vi "Begin.vi"(8 "error in":errorcluster) -> (0 "error out":errorcluster)   [LabVIEW 2020]
doc: "Called before other user functions, this VI is expected to open initial I/O refnums, load in file data, and do all program initialization. Notice that the <B>error out</B> terminal is simply used for data flow. Wiring it to other structures or subVIs ensures that this VI runs first."
uses:
  <vilib>/Rock Robotics/WPI/DriverStation/WPI_DriverStationRobotMode2.ctl
  <vilib>/Rock Robotics/WPI/Joystick/WPI_JoystickDeviceEnum.ctl
  <vilib>/Rock Robotics/SystemInterfaces/i2clib/i2c_bus.ctl
  <vilib>/Rock Robotics/WPI/Solenoid/WPI_SolenoidChannel.ctl
  <vilib>/Rock Robotics/SystemInterfaces/DIO/FPGA_DIOChannel.ctl
  <vilib>/Rock Robotics/WPI/ThirdParty/Phoenix-LabVIEW/Motor Controller/Controls/CTRE_Phoenix_MotorControl_StatusFrameEnhanced.ctl
  Robot Global Data.vi
  <vilib>/Rock Robotics/Network Tables/NT Write String Array.vi
  <vilib>/Rock Robotics/WPI/Solenoid/WPI_SolenoidOpenDouble.vi
  <vilib>/Rock Robotics/WPI/Switch/WPI_SwitchOpenLimit.vi
  <vilib>/Rock Robotics/WPI/Switch/WPI_SwitchOpenCounting.vi
  <vilib>/Rock Robotics/WPI/ThirdParty/Phoenix-LabVIEW/Motor Controller/Get/CTRE_Phoenix_MotorController_GetSelectedSensorData.vi
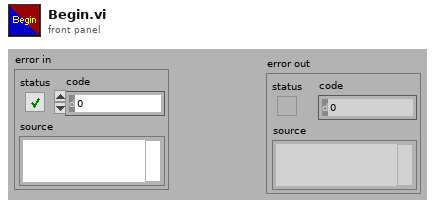
[diagram p1: front panel]
types:
  T1 = typedef "CTRE_Phoenix_MotorControl_StatusFrameEnhanced.ctl" = u16
  T2 = typedef "FPGA_DIOChannel.ctl" = enum8{"DIO 0", "DIO 1", "DIO 2", "DIO 3", "DIO 4", "DIO 5", "DIO 6", "DIO 7", "DIO 8", "DIO 9", "DIO MXP 0", "DIO MXP 1", "DIO MXP 2", "DIO MXP 3", "DIO MXP 4", "DIO MXP 5", "DIO MXP 6", "DIO MXP 7", "DIO MXP 8", "DIO MXP 9", "DIO MXP 10", "DIO MXP 11", "DIO MXP 12", "DIO MXP 13", "DIO MXP 14", "DIO MXP 15", "SPI Port CS1", "SPI Port CS2", "SPI Port CS3", "SPI Port MISO", "SPI Port MOSI", "Invalid"}
  T3 = typedef "WPI_SolenoidChannel.ctl" = enum8{"Solenoid 0", "Solenoid 1", "Solenoid 2", "Solenoid 3", "Solenoid 4", "Solenoid 5", "Solenoid 6", "Solenoid 7", "Solenoid 8", "Solenoid 9", "Solenoid 10", "Solenoid 11", "Solenoid 12", "Solenoid 13", "Solenoid 14", "Solenoid 15", "Invalid"}
  T4 = typedef "i2c_bus.ctl" = enum16{"I2C On-Board", "I2C MXP", "Invalid"}
  T5 = typedef "WPI_JoystickDeviceEnum.ctl" = enum16{"USB 0", "USB 1", "USB 2", "USB 3", "USB 4", "USB 5"}
  T6 = typedef "WPI_DriverStationRobotMode2.ctl" = enum16{"Autonomous Disabled", "Autonomous Enabled", "Teleop Disabled", "Teleop Enabled", "Disconnected", "Finish", "Test Disabled", "Test Enabled", "Emergency Stopped"}
  T7 = typedef "WPI_JoystickDevRef.ctl" = cluster{"Device":T5}
  T8 = typedef "WPI_CompressorDevRef.ctl" = cluster{"DevStatus":errorcluster, "Pneumatics Control Module":u8}
  T9 = typedef "WPI_SolenoidDevRef.ctl" = cluster{"DevStatus":errorcluster, "Pneumatics Control Module":u8, "Forward Solenoid Channel":T3, "Reverse Solenoid Channel":T3}
  T10 = typedef "WPI_SwitchDevRef.ctl" = cluster{"DevStatus":errorcluster, "DIO Channel":T2, "CntIndex":T11, "Normally Closed":bool}
  T11 = typedef "FPGA_CounterCtrSystemIndex.ctl" = enum8{"Ctr 0", "Ctr 1", "Ctr 2", "Ctr 3", "Ctr 4", "Ctr 5", "Ctr 6", "Ctr 7", "Invalid"}
  T12 = typedef "WPI_MotorControlDeviceRef.ctl" = cluster{"DeviceStatus":errorcluster, "Type":T13, "PWM":cluster{"PWM Channel":T14, "DeadBand":T15}, "CAN":cluster{"Device Number":u8, "SetOutput VI Ref":variant, "GetOutput VI Ref":variant, "Enable VI Ref":variant, "Disable VI Ref":variant, "Data":variant}, "Invert":bool, "DIO PWM":cluster{"PWM \"Enable\" Channel":T14, "DIOChannel":T2, "PWM Rate":dbl}}
  T13 = typedef "WPI_MotorControlType.ctl" = enum16{"PWM", "CAN", "DIO PWM"}
  T14 = typedef "FPGA_DIOPWMChannel.ctl" = enum8{"PWM 0", "PWM 1", "PWM 2", "PWM 3", "PWM 4", "PWM 5", "PWM 6", "PWM 7", "PWM 8", "PWM 9", "PWM MXP 0", "PWM MXP 1", "PWM MXP 2", "PWM MXP 3", "PWM MXP 4", "PWM MXP 5", "PWM MXP 6", "PWM MXP 7", "PWM MXP 8", "PWM MXP 9", "Invalid"}
  T15 = typedef "WPI_PWMDeadband.ctl" = cluster{"Name":string, "maxPositivePwm":i32, "minPositivePwm":i32, "centerPwm":i32, "maxNegativePwm":i32, "minNegativePwm":i32, "angularRange":u16}
  T16 = typedef "Color Sensor V3 DevRef.ctl" = cluster{"I2CDevRef":T17}
  T17 = typedef "WPI_I2CDevRef.ctl" = cluster{"DevStatus":errorcluster, "Device Address":u8, "Handle":i32, "I2C Bus":T4}
  T18 = typedef "CTRE_PigeonIMU_DeviceRef.ctl" = cluster{"DeviceStatus":errorcluster, "Device Number":u8, "Type":T19, "Device ID":u32, "Handle":u64, "UsageFrame":u32, "Library Path":path}
  T19 = typedef "CTRE_PigeonIMU_ConnectionType.ctl" = u32
  T20 = typedef "CTRE_Phoenix_CANcoder_DeviceRef.ctl" = cluster{"DeviceStatus":errorcluster, "Device Number":u8, "Handle":u64, "UsageFrame":u32, "Library Path":path}
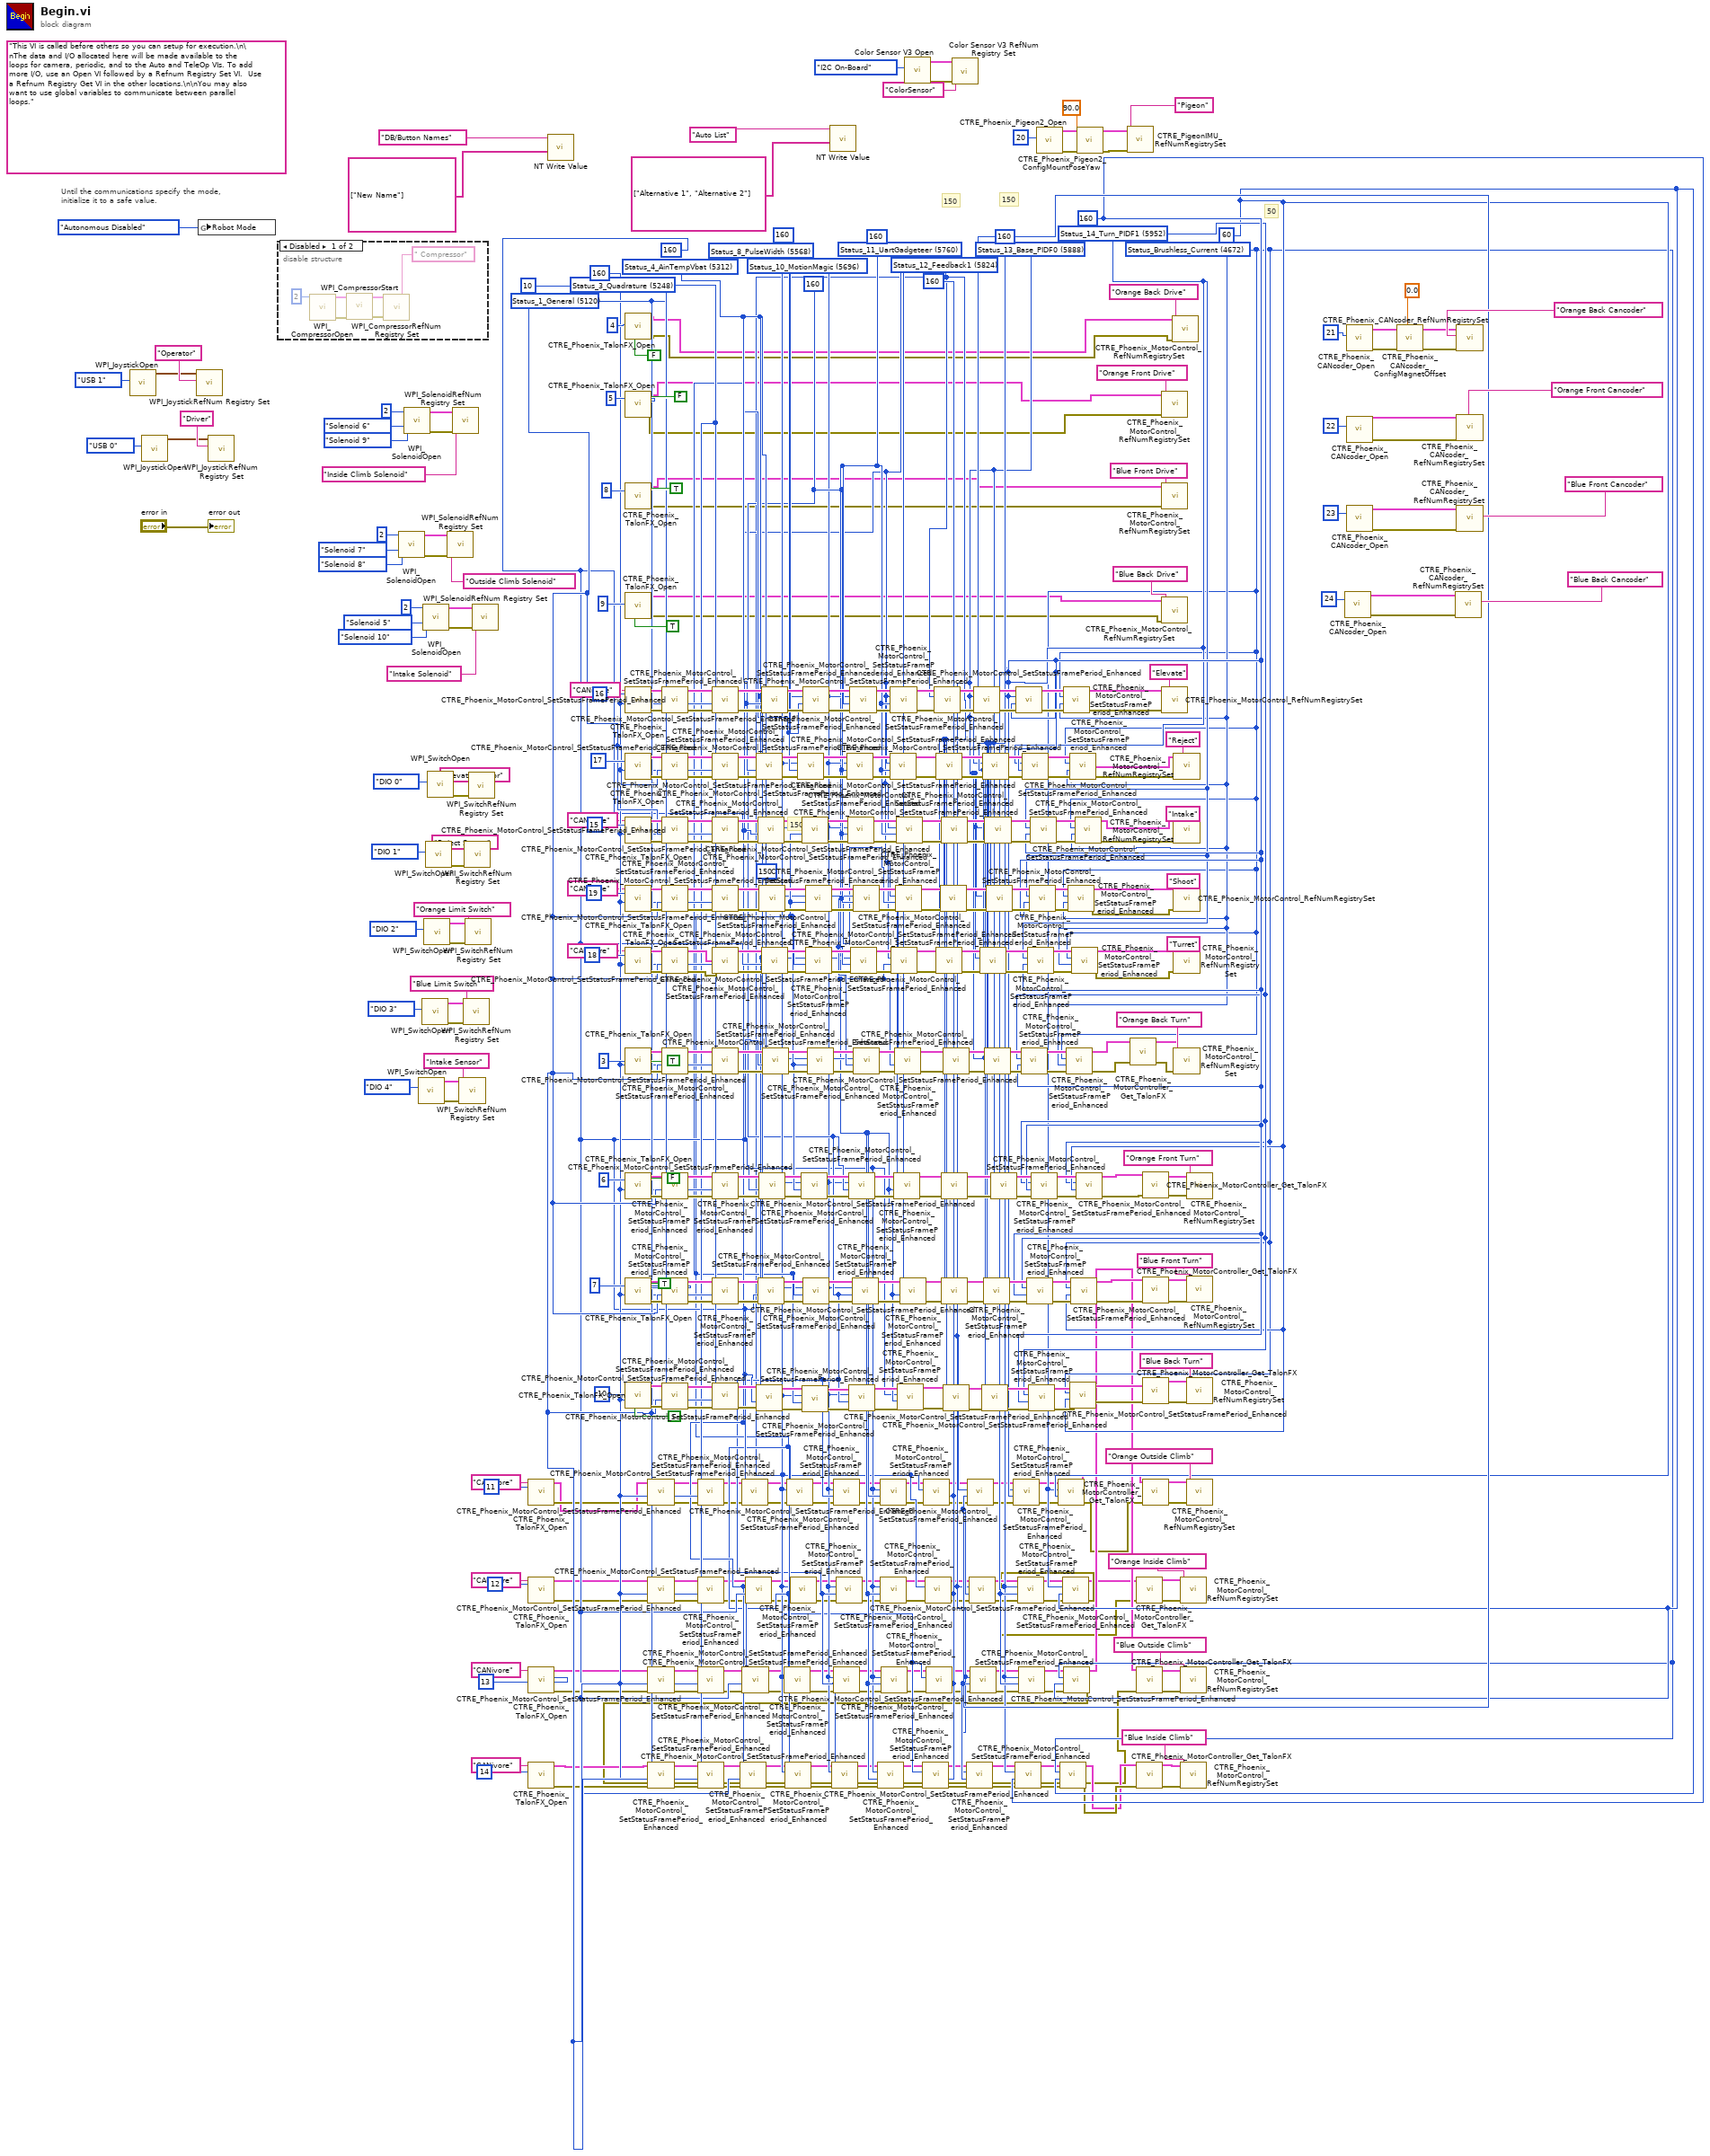
[diagram p0: block diagram]
diagram:
  w122 = 60 ("periodMs")
  w121 = T1 4672 items=["Status_1_General"=5120, "Status_2_Feedback0"=5184, "Status_3_Quadrature"=5248, "Status_4_AinTempVbat"=5312, "Status_6_Misc"=5440, "Status_7_CommStatus"=5504, "Status_8_PulseWidth"=5568, "Status_9_MotProfBuffer"=5632, "Status_10_MotionMagic"=5696, "Status_11_UartGadgeteer"=5760, "Status_12_Feedback1"=5824, "Status_13_Base_PIDF0"=5888, "Status_14_Turn_PIDF1"=5952, "Status_15_FirmwareApiStatus"=6016, "Status_Brushless_Current"=4672] ("Status Frame")
  w124 = 160 ("periodMs")
  w123 = T1 5952 items=["Status_1_General"=5120, "Status_2_Feedback0"=5184, "Status_3_Quadrature"=5248, "Status_4_AinTempVbat"=5312, "Status_6_Misc"=5440, "Status_7_CommStatus"=5504, "Status_8_PulseWidth"=5568, "Status_9_MotProfBuffer"=5632, "Status_10_MotionMagic"=5696, "Status_11_UartGadgeteer"=5760, "Status_12_Feedback1"=5824, "Status_13_Base_PIDF0"=5888, "Status_14_Turn_PIDF1"=5952, "Status_15_FirmwareApiStatus"=6016, "Status_Brushless_Current"=4672] ("Status Frame")
  w126 = 160 ("periodMs")
  w125 = T1 5888 items=["Status_1_General"=5120, "Status_2_Feedback0"=5184, "Status_3_Quadrature"=5248, "Status_4_AinTempVbat"=5312, "Status_6_Misc"=5440, "Status_7_CommStatus"=5504, "Status_8_PulseWidth"=5568, "Status_9_MotProfBuffer"=5632, "Status_10_MotionMagic"=5696, "Status_11_UartGadgeteer"=5760, "Status_12_Feedback1"=5824, "Status_13_Base_PIDF0"=5888, "Status_14_Turn_PIDF1"=5952, "Status_15_FirmwareApiStatus"=6016, "Status_Brushless_Current"=4672] ("Status Frame")
  w128 = 160 ("periodMs")
  w127 = T1 5824 items=["Status_1_General"=5120, "Status_2_Feedback0"=5184, "Status_3_Quadrature"=5248, "Status_4_AinTempVbat"=5312, "Status_6_Misc"=5440, "Status_7_CommStatus"=5504, "Status_8_PulseWidth"=5568, "Status_9_MotProfBuffer"=5632, "Status_10_MotionMagic"=5696, "Status_11_UartGadgeteer"=5760, "Status_12_Feedback1"=5824, "Status_13_Base_PIDF0"=5888, "Status_14_Turn_PIDF1"=5952, "Status_15_FirmwareApiStatus"=6016, "Status_Brushless_Current"=4672] ("Status Frame")
  w132 = 160 ("periodMs")
  w131 = T1 5760 items=["Status_1_General"=5120, "Status_2_Feedback0"=5184, "Status_3_Quadrature"=5248, "Status_4_AinTempVbat"=5312, "Status_6_Misc"=5440, "Status_7_CommStatus"=5504, "Status_8_PulseWidth"=5568, "Status_9_MotProfBuffer"=5632, "Status_10_MotionMagic"=5696, "Status_11_UartGadgeteer"=5760, "Status_12_Feedback1"=5824, "Status_13_Base_PIDF0"=5888, "Status_14_Turn_PIDF1"=5952, "Status_15_FirmwareApiStatus"=6016, "Status_Brushless_Current"=4672] ("Status Frame")
  w241 = T1 5696 items=["Status_1_General"=5120, "Status_2_Feedback0"=5184, "Status_3_Quadrature"=5248, "Status_4_AinTempVbat"=5312, "Status_6_Misc"=5440, "Status_7_CommStatus"=5504, "Status_8_PulseWidth"=5568, "Status_9_MotProfBuffer"=5632, "Status_10_MotionMagic"=5696, "Status_11_UartGadgeteer"=5760, "Status_12_Feedback1"=5824, "Status_13_Base_PIDF0"=5888, "Status_14_Turn_PIDF1"=5952, "Status_15_FirmwareApiStatus"=6016, "Status_Brushless_Current"=4672] ("Status Frame")
  w242 = 160 ("periodMs")
  w262 = 160 ("periodMs")
  w261 = T1 5568 items=["Status_1_General"=5120, "Status_2_Feedback0"=5184, "Status_3_Quadrature"=5248, "Status_4_AinTempVbat"=5312, "Status_6_Misc"=5440, "Status_7_CommStatus"=5504, "Status_8_PulseWidth"=5568, "Status_9_MotProfBuffer"=5632, "Status_10_MotionMagic"=5696, "Status_11_UartGadgeteer"=5760, "Status_12_Feedback1"=5824, "Status_13_Base_PIDF0"=5888, "Status_14_Turn_PIDF1"=5952, "Status_15_FirmwareApiStatus"=6016, "Status_Brushless_Current"=4672] ("Status Frame")
  w282 = 160 ("periodMs")
  w281 = T1 5312 items=["Status_1_General"=5120, "Status_2_Feedback0"=5184, "Status_3_Quadrature"=5248, "Status_4_AinTempVbat"=5312, "Status_6_Misc"=5440, "Status_7_CommStatus"=5504, "Status_8_PulseWidth"=5568, "Status_9_MotProfBuffer"=5632, "Status_10_MotionMagic"=5696, "Status_11_UartGadgeteer"=5760, "Status_12_Feedback1"=5824, "Status_13_Base_PIDF0"=5888, "Status_14_Turn_PIDF1"=5952, "Status_15_FirmwareApiStatus"=6016, "Status_Brushless_Current"=4672] ("Status Frame")
  w302 = 160 ("periodMs")
  w301 = T1 5248 items=["Status_1_General"=5120, "Status_2_Feedback0"=5184, "Status_3_Quadrature"=5248, "Status_4_AinTempVbat"=5312, "Status_6_Misc"=5440, "Status_7_CommStatus"=5504, "Status_8_PulseWidth"=5568, "Status_9_MotProfBuffer"=5632, "Status_10_MotionMagic"=5696, "Status_11_UartGadgeteer"=5760, "Status_12_Feedback1"=5824, "Status_13_Base_PIDF0"=5888, "Status_14_Turn_PIDF1"=5952, "Status_15_FirmwareApiStatus"=6016, "Status_Brushless_Current"=4672] ("Status Frame")
  w304 = 10 ("periodMs")
  w303 = T1 5120 items=["Status_1_General"=5120, "Status_2_Feedback0"=5184, "Status_3_Quadrature"=5248, "Status_4_AinTempVbat"=5312, "Status_6_Misc"=5440, "Status_7_CommStatus"=5504, "Status_8_PulseWidth"=5568, "Status_9_MotProfBuffer"=5632, "Status_10_MotionMagic"=5696, "Status_11_UartGadgeteer"=5760, "Status_12_Feedback1"=5824, "Status_13_Base_PIDF0"=5888, "Status_14_Turn_PIDF1"=5952, "Status_15_FirmwareApiStatus"=6016, "Status_Brushless_Current"=4672] ("Status Frame")
  (unwired) "This VI is called before others so you can setup for execution.\n\nThe data and I/O allocated here will be made available to the loops for camera, periodic, and to the Auto and TeleOp VIs. To add more I/O, use an Open VI followed by a Refnum Registry Set VI.  Use a Refnum Registry Get VI in the other locations.\n\nYou may also want to use global variables to communicate between parallel loops."
  # "50"
  # "150"
  # "150"
  # "150"
  # "Until the communications specify the mode,\ninitialize it to a safe value."
  n1 = call <vilib>:"WPI_JoystickOpen.vi"("JoystickDevice"=WPI_JoystickDeviceEnum."USB 1") -> ("JoystickDevRef"=w451:T7)  [unwired: 10 in]
  n2 = call <vilib>:"WPI_JoystickOpen.vi"("JoystickDevice"=WPI_JoystickDeviceEnum."USB 0") -> ("JoystickDevRef"=w459:T7)  [unwired: 10 in]
  n3 = call <vilib>:"WPI_JoystickRefNum Registry Set.vi"("refnum name"="Operator", "JoystickDevRef"=w451) -> ()  [unwired: 8 in, 2 out]
  n4 = global write "Robot Global Data.vi" "Robot Mode"(WPI_DriverStationRobotMode2."Autonomous Disabled" ("Robot Mode")) -> ()
  n5 = call <vilib>:"WPI_JoystickRefNum Registry Set.vi"("refnum name"="Driver", "JoystickDevRef"=w459) -> ()  [unwired: 8 in, 2 out]
  n6 = disable-structure shown="Disabled" {
    frame Disabled {
      n7 = call <vilib>:"WPI_CompressorOpen.vi"("Pneumatics device (def)"=u8 2) -> ("CompressorDevRef"=w466:T8, "error out"=w467:errorcluster)  [unwired: 13 in]
      n8 = call <vilib>:"WPI_CompressorStart.vi"("error in (no error)"=w467, "CompressorDevRef"=w466) -> ("error out"=w465:errorcluster, "CompressorDevRef"=w464:T8)  [unwired: 8 in]
      n9 = call <vilib>:"WPI_CompressorRefNum Registry Set.vi"("error in (no error)"=w465, "refnum name"=" Compressor", "CompressorDevRef"=w464) -> ()  [unwired: 7 in, 2 out]
    }
    frame Enabled {
    }
  }
  n10 = call-poly <vilib>:"WPI_SolenoidOpen.vi"("Reverse Solenoid Channel"=WPI_SolenoidChannel."Solenoid 8", "Forward Solenoid Channel"=WPI_SolenoidChannel."Solenoid 7", "Pneumatics Device (def)"=u8 2) -> ("error out"=w405:errorcluster, "SolenoidDevRef"=w404:T9)  [unwired: 7 in]
  n11 = call-poly <vilib>:"WPI_SolenoidOpen.vi"("Reverse Solenoid Channel"=WPI_SolenoidChannel."Solenoid 9", "Forward Solenoid Channel"=WPI_SolenoidChannel."Solenoid 6", "Pneumatics Device (def)"=u8 2) -> ("error out"=w408:errorcluster, "SolenoidDevRef"=w407:T9)  [unwired: 7 in]
  n12 = call-poly <vilib>:"WPI_SwitchOpen.vi"("DIO Channel"=FPGA_DIOChannel."DIO 4") -> ("error out"=w365:errorcluster, "SwitchDevRef"=w364:T10)  [unwired: 9 in]
  n13 = call-poly <vilib>:"WPI_SwitchOpen.vi"("DIO Channel"=FPGA_DIOChannel."DIO 3") -> ("error out"=w369:errorcluster, "SwitchDevRef"=w368:T10)  [unwired: 9 in]
  n14 = call-poly <vilib>:"WPI_SolenoidOpen.vi"("Reverse Solenoid Channel"=WPI_SolenoidChannel."Solenoid 10", "Forward Solenoid Channel"=WPI_SolenoidChannel."Solenoid 5", "Pneumatics Device (def)"=u8 2) -> ("error out"=w402:errorcluster, "SolenoidDevRef"=w401:T9)  [unwired: 7 in]
  n15 = call-poly <vilib>:"WPI_SwitchOpen.vi"("DIO Channel"=FPGA_DIOChannel."DIO 2") -> ("error out"=w373:errorcluster, "SwitchDevRef"=w372:T10)  [unwired: 9 in]
  n16 = call-poly <vilib>:"WPI_SwitchOpen.vi"("DIO Channel"=FPGA_DIOChannel."DIO 1") -> ("error out"=w386:errorcluster, "SwitchDevRef"=w385:T10)  [unwired: 9 in]
  n17 = call-poly <vilib>:"WPI_SwitchOpen.vi"("DIO Channel"=FPGA_DIOChannel."DIO 0") -> ("error out"=w390:errorcluster, "SwitchDevRef"=w389:T10)  [unwired: 9 in]
  n18 = call <vilib>:"WPI_SolenoidRefNum Registry Set.vi"("error in (no error)"=w405, "refnum name"="Outside Climb Solenoid", "SolenoidDevRef"=w404) -> ()  [unwired: 7 in, 2 out]
  n19 = call <vilib>:"WPI_SolenoidRefNum Registry Set.vi"("error in (no error)"=w408, "refnum name"="Inside Climb Solenoid", "SolenoidDevRef"=w407) -> ()  [unwired: 7 in, 2 out]
  n20 = call <vilib>:"WPI_SwitchRefNum Registry Set.vi"("error in (no error)"=w365, "refnum name"="Intake Sensor", "SwitchDevRef"=w364) -> ()  [unwired: 7 in, 2 out]
  n21 = call <vilib>:"WPI_SwitchRefNum Registry Set.vi"("error in (no error)"=w369, "refnum name"="Blue Limit Switch", "SwitchDevRef"=w368) -> ()  [unwired: 7 in, 2 out]
  n22 = call <vilib>:"WPI_SwitchRefNum Registry Set.vi"("error in (no error)"=w386, "refnum name"="Reject Sensor", "SwitchDevRef"=w385) -> ()  [unwired: 7 in, 2 out]
  n23 = call <vilib>:"WPI_SwitchRefNum Registry Set.vi"("error in (no error)"=w373, "refnum name"="Orange Limit Switch", "SwitchDevRef"=w372) -> ()  [unwired: 7 in, 2 out]
  n24 = call <vilib>:"WPI_SwitchRefNum Registry Set.vi"("error in (no error)"=w390, "refnum name"="Elevate Sensor", "SwitchDevRef"=w389) -> ()  [unwired: 7 in, 2 out]
  n25 = call <vilib>:"WPI_SolenoidRefNum Registry Set.vi"("error in (no error)"=w402, "refnum name"="Intake Solenoid", "SolenoidDevRef"=w401) -> ()  [unwired: 7 in, 2 out]
  n26 = call <vilib>:"CTRE_Phoenix_TalonFX_Open.vi"("Device Number"=u8 11, "CAN Bus"="CANivore") -> ("error out"=w27:errorcluster, "PhoenixMotorControlDevRef"=w26:T12)  [unwired: 8 in]
  n27 = call <vilib>:"CTRE_Phoenix_TalonFX_Open.vi"("Device Number"=u8 12, "CAN Bus"="CANivore") -> ("error out"=w29:errorcluster, "PhoenixMotorControlDevRef"=w28:T12)  [unwired: 8 in]
  n28 = call <vilib>:"CTRE_Phoenix_TalonFX_Open.vi"("Device Number"=u8 13, "CAN Bus"="CANivore") -> ("error out"=w31:errorcluster, "PhoenixMotorControlDevRef"=w30:T12)  [unwired: 8 in]
  n29 = call <vilib>:"CTRE_Phoenix_TalonFX_Open.vi"("Device Number"=u8 14, "CAN Bus"="CANivore") -> ("error out"=w33:errorcluster, "PhoenixMotorControlDevRef"=w32:T12)  [unwired: 8 in]
  n30 = call-poly <vilib>:"NT Write Value.vi"("String Array"=string[] ["New Name"], "Name"="DB/Button Names") -> ()  [unwired: 9 in, 1 out]
  n31 = call <vilib>:"CTRE_Phoenix_TalonFX_Open.vi"("Invert"=FALSE, "Device Number"=u8 4) -> ("error out"=w114:errorcluster, "PhoenixMotorControlDevRef"=w113:T12)  [unwired: 8 in]
  n32 = call <vilib>:"CTRE_Phoenix_TalonFX_Open.vi"("Invert"=FALSE, "Device Number"=u8 5) -> ("error out"=w116:errorcluster, "PhoenixMotorControlDevRef"=w115:T12)  [unwired: 8 in]
  n33 = call <vilib>:"CTRE_Phoenix_TalonFX_Open.vi"("Invert"=TRUE, "Device Number"=u8 8) -> ("error out"=w111:errorcluster, "PhoenixMotorControlDevRef"=w112:T12)  [unwired: 8 in]
  n34 = call <vilib>:"CTRE_Phoenix_TalonFX_Open.vi"("Invert"=TRUE, "Device Number"=u8 9) -> ("error out"=w109:errorcluster, "PhoenixMotorControlDevRef"=w110:T12)  [unwired: 8 in]
  n35 = call <vilib>:"CTRE_Phoenix_TalonFX_Open.vi"("Device Number"=u8 16, "CAN Bus"="CANivore") -> ("error out"=w345:errorcluster, "PhoenixMotorControlDevRef"=w344:T12)  [unwired: 8 in]
  n36 = call <vilib>:"CTRE_Phoenix_TalonFX_Open.vi"("Device Number"=u8 17) -> ("error out"=w343:errorcluster, "PhoenixMotorControlDevRef"=w342:T12)  [unwired: 9 in]
  n37 = call <vilib>:"CTRE_Phoenix_TalonFX_Open.vi"("Device Number"=u8 15, "CAN Bus"="CANivore") -> ("error out"=w341:errorcluster, "PhoenixMotorControlDevRef"=w340:T12)  [unwired: 8 in]
  n38 = call <vilib>:"CTRE_Phoenix_TalonFX_Open.vi"("Device Number"=u8 19, "CAN Bus"="CANivore") -> ("error out"=w339:errorcluster, "PhoenixMotorControlDevRef"=w338:T12)  [unwired: 8 in]
  n39 = call <vilib>:"CTRE_Phoenix_TalonFX_Open.vi"("Device Number"=u8 18, "CAN Bus"="CANivore") -> ("error out"=w337:errorcluster, "PhoenixMotorControlDevRef"=w336:T12)  [unwired: 8 in]
  n40 = call <vilib>:"CTRE_Phoenix_TalonFX_Open.vi"("Invert"=TRUE, "Device Number"=u8 3) -> ("error out"=w325:errorcluster, "PhoenixMotorControlDevRef"=w324:T12)  [unwired: 8 in]
  n41 = call <vilib>:"CTRE_Phoenix_TalonFX_Open.vi"("Invert"=FALSE, "Device Number"=u8 6) -> ("error out"=w323:errorcluster, "PhoenixMotorControlDevRef"=w322:T12)  [unwired: 8 in]
  n42 = call <vilib>:"CTRE_Phoenix_TalonFX_Open.vi"("Invert"=TRUE, "Device Number"=u8 7) -> ("error out"=w321:errorcluster, "PhoenixMotorControlDevRef"=w320:T12)  [unwired: 8 in]
  n43 = call <vilib>:"CTRE_Phoenix_TalonFX_Open.vi"("Invert"=FALSE, "Device Number"=u8 10) -> ("error out"=w319:errorcluster, "PhoenixMotorControlDevRef"=w318:T12)  [unwired: 8 in]
  n44 = call <vilib>:"CTRE_Phoenix_MotorControl_SetStatusFramePeriod_Enhanced.vi"("error in (no error)"=w27, "periodMs"=w304, "Status Frame"=w303, "PhoenixMotorControlDevRef"=w26) -> ("error out"=w40:errorcluster, "PhoenixMotorControlDevRef"=w17:T12)  [unwired: 6 in]
  n45 = call <vilib>:"CTRE_Phoenix_MotorControl_SetStatusFramePeriod_Enhanced.vi"("error in (no error)"=w29, "periodMs"=w304, "Status Frame"=w303, "PhoenixMotorControlDevRef"=w28) -> ("error out"=w38:errorcluster, "PhoenixMotorControlDevRef"=w39:T12)  [unwired: 6 in]
  n46 = call <vilib>:"CTRE_Phoenix_MotorControl_SetStatusFramePeriod_Enhanced.vi"("error in (no error)"=w31, "periodMs"=w304, "Status Frame"=w303, "PhoenixMotorControlDevRef"=w30) -> ("error out"=w36:errorcluster, "PhoenixMotorControlDevRef"=w37:T12)  [unwired: 6 in]
  n47 = call <vilib>:"CTRE_Phoenix_MotorControl_SetStatusFramePeriod_Enhanced.vi"("error in (no error)"=w33, "periodMs"=w304, "Status Frame"=w303, "PhoenixMotorControlDevRef"=w32) -> ("error out"=w34:errorcluster, "PhoenixMotorControlDevRef"=w35:T12)  [unwired: 6 in]
  n48 = call <vilib>:"CTRE_Phoenix_MotorControl_SetStatusFramePeriod_Enhanced.vi"("error in (no error)"=w345, "periodMs"=w304, "Status Frame"=w303, "PhoenixMotorControlDevRef"=w344) -> ("error out"=w327:errorcluster, "PhoenixMotorControlDevRef"=w326:T12)  [unwired: 6 in]
  n49 = call <vilib>:"CTRE_Phoenix_MotorControl_SetStatusFramePeriod_Enhanced.vi"("error in (no error)"=w343, "periodMs"=w304, "Status Frame"=w303, "PhoenixMotorControlDevRef"=w342) -> ("error out"=w329:errorcluster, "PhoenixMotorControlDevRef"=w328:T12)  [unwired: 6 in]
  n50 = call <vilib>:"CTRE_Phoenix_MotorControl_SetStatusFramePeriod_Enhanced.vi"("error in (no error)"=w341, "periodMs"=w304, "Status Frame"=w303, "PhoenixMotorControlDevRef"=w340) -> ("error out"=w331:errorcluster, "PhoenixMotorControlDevRef"=w330:T12)  [unwired: 6 in]
  n51 = call <vilib>:"CTRE_Phoenix_MotorControl_SetStatusFramePeriod_Enhanced.vi"("error in (no error)"=w339, "periodMs"=w304, "Status Frame"=w303, "PhoenixMotorControlDevRef"=w338) -> ("error out"=w333:errorcluster, "PhoenixMotorControlDevRef"=w332:T12)  [unwired: 6 in]
  n52 = call <vilib>:"CTRE_Phoenix_MotorControl_SetStatusFramePeriod_Enhanced.vi"("error in (no error)"=w337, "periodMs"=w304, "Status Frame"=w303, "PhoenixMotorControlDevRef"=w336) -> ("error out"=w335:errorcluster, "PhoenixMotorControlDevRef"=w334:T12)  [unwired: 6 in]
  n53 = call <vilib>:"CTRE_Phoenix_MotorControl_SetStatusFramePeriod_Enhanced.vi"("error in (no error)"=w325, "periodMs"=w304, "Status Frame"=w303, "PhoenixMotorControlDevRef"=w324) -> ("error out"=w311:errorcluster, "PhoenixMotorControlDevRef"=w310:T12)  [unwired: 6 in]
  n54 = call <vilib>:"CTRE_Phoenix_MotorControl_SetStatusFramePeriod_Enhanced.vi"("error in (no error)"=w323, "periodMs"=w304, "Status Frame"=w303, "PhoenixMotorControlDevRef"=w322) -> ("error out"=w313:errorcluster, "PhoenixMotorControlDevRef"=w312:T12)  [unwired: 6 in]
  n55 = call <vilib>:"CTRE_Phoenix_MotorControl_SetStatusFramePeriod_Enhanced.vi"("error in (no error)"=w321, "periodMs"=w304, "Status Frame"=w303, "PhoenixMotorControlDevRef"=w320) -> ("error out"=w315:errorcluster, "PhoenixMotorControlDevRef"=w314:T12)  [unwired: 6 in]
  n56 = call <vilib>:"CTRE_Phoenix_MotorControl_SetStatusFramePeriod_Enhanced.vi"("error in (no error)"=w319, "periodMs"=w304, "Status Frame"=w303, "PhoenixMotorControlDevRef"=w318) -> ("error out"=w317:errorcluster, "PhoenixMotorControlDevRef"=w316:T12)  [unwired: 6 in]
  n57 = call <vilib>:"CTRE_Phoenix_MotorControl_SetStatusFramePeriod_Enhanced.vi"("error in (no error)"=w40, "periodMs"=w302, "Status Frame"=w301, "PhoenixMotorControlDevRef"=w17) -> ("error out"=w41:errorcluster, "PhoenixMotorControlDevRef"=w16:T12)  [unwired: 6 in]
  n58 = call <vilib>:"CTRE_Phoenix_MotorControl_SetStatusFramePeriod_Enhanced.vi"("error in (no error)"=w38, "periodMs"=w302, "Status Frame"=w301, "PhoenixMotorControlDevRef"=w39) -> ("error out"=w42:errorcluster, "PhoenixMotorControlDevRef"=w43:T12)  [unwired: 6 in]
  n59 = call <vilib>:"CTRE_Phoenix_MotorControl_SetStatusFramePeriod_Enhanced.vi"("error in (no error)"=w36, "periodMs"=w302, "Status Frame"=w301, "PhoenixMotorControlDevRef"=w37) -> ("error out"=w44:errorcluster, "PhoenixMotorControlDevRef"=w45:T12)  [unwired: 6 in]
  n60 = call <vilib>:"CTRE_Phoenix_MotorControl_SetStatusFramePeriod_Enhanced.vi"("error in (no error)"=w34, "periodMs"=w302, "Status Frame"=w301, "PhoenixMotorControlDevRef"=w35) -> ("error out"=w46:errorcluster, "PhoenixMotorControlDevRef"=w47:T12)  [unwired: 6 in]
  n61 = call <vilib>:"CTRE_Phoenix_MotorControl_SetStatusFramePeriod_Enhanced.vi"("error in (no error)"=w327, "periodMs"=w302, "Status Frame"=w301, "PhoenixMotorControlDevRef"=w326) -> ("error out"=w300:errorcluster, "PhoenixMotorControlDevRef"=w299:T12)  [unwired: 6 in]
  n62 = call <vilib>:"CTRE_Phoenix_MotorControl_SetStatusFramePeriod_Enhanced.vi"("error in (no error)"=w329, "periodMs"=w302, "Status Frame"=w301, "PhoenixMotorControlDevRef"=w328) -> ("error out"=w298:errorcluster, "PhoenixMotorControlDevRef"=w297:T12)  [unwired: 6 in]
  n63 = call <vilib>:"CTRE_Phoenix_MotorControl_SetStatusFramePeriod_Enhanced.vi"("error in (no error)"=w331, "periodMs"=w302, "Status Frame"=w301, "PhoenixMotorControlDevRef"=w330) -> ("error out"=w296:errorcluster, "PhoenixMotorControlDevRef"=w295:T12)  [unwired: 6 in]
  n64 = call <vilib>:"CTRE_Phoenix_MotorControl_SetStatusFramePeriod_Enhanced.vi"("error in (no error)"=w333, "periodMs"=w302, "Status Frame"=w301, "PhoenixMotorControlDevRef"=w332) -> ("error out"=w294:errorcluster, "PhoenixMotorControlDevRef"=w293:T12)  [unwired: 6 in]
  n65 = call <vilib>:"CTRE_Phoenix_MotorControl_SetStatusFramePeriod_Enhanced.vi"("error in (no error)"=w335, "periodMs"=w302, "Status Frame"=w301, "PhoenixMotorControlDevRef"=w334) -> ("error out"=w292:errorcluster, "PhoenixMotorControlDevRef"=w291:T12)  [unwired: 6 in]
  n66 = call <vilib>:"CTRE_Phoenix_MotorControl_SetStatusFramePeriod_Enhanced.vi"("error in (no error)"=w311, "periodMs"=w302, "Status Frame"=w301, "PhoenixMotorControlDevRef"=w310) -> ("error out"=w290:errorcluster, "PhoenixMotorControlDevRef"=w289:T12)  [unwired: 6 in]
  n67 = call <vilib>:"CTRE_Phoenix_MotorControl_SetStatusFramePeriod_Enhanced.vi"("error in (no error)"=w313, "periodMs"=w302, "Status Frame"=w301, "PhoenixMotorControlDevRef"=w312) -> ("error out"=w288:errorcluster, "PhoenixMotorControlDevRef"=w287:T12)  [unwired: 6 in]
  n68 = call <vilib>:"CTRE_Phoenix_MotorControl_SetStatusFramePeriod_Enhanced.vi"("error in (no error)"=w315, "periodMs"=w302, "Status Frame"=w301, "PhoenixMotorControlDevRef"=w314) -> ("error out"=w286:errorcluster, "PhoenixMotorControlDevRef"=w285:T12)  [unwired: 6 in]
  n69 = call <vilib>:"CTRE_Phoenix_MotorControl_SetStatusFramePeriod_Enhanced.vi"("error in (no error)"=w317, "periodMs"=w302, "Status Frame"=w301, "PhoenixMotorControlDevRef"=w316) -> ("error out"=w284:errorcluster, "PhoenixMotorControlDevRef"=w283:T12)  [unwired: 6 in]
  n70 = call <vilib>:"CTRE_Phoenix_MotorControl_SetStatusFramePeriod_Enhanced.vi"("error in (no error)"=w46, "periodMs"=w282, "Status Frame"=w281, "PhoenixMotorControlDevRef"=w47) -> ("error out"=w53:errorcluster, "PhoenixMotorControlDevRef"=w54:T12)  [unwired: 6 in]
  n71 = call <vilib>:"CTRE_Phoenix_MotorControl_SetStatusFramePeriod_Enhanced.vi"("error in (no error)"=w41, "periodMs"=w282, "Status Frame"=w281, "PhoenixMotorControlDevRef"=w16) -> ("error out"=w48:errorcluster, "PhoenixMotorControlDevRef"=w15:T12)  [unwired: 6 in]
  n72 = call <vilib>:"CTRE_Phoenix_MotorControl_SetStatusFramePeriod_Enhanced.vi"("error in (no error)"=w44, "periodMs"=w282, "Status Frame"=w281, "PhoenixMotorControlDevRef"=w45) -> ("error out"=w51:errorcluster, "PhoenixMotorControlDevRef"=w52:T12)  [unwired: 6 in]
  n73 = call <vilib>:"CTRE_Phoenix_MotorControl_SetStatusFramePeriod_Enhanced.vi"("error in (no error)"=w42, "periodMs"=w282, "Status Frame"=w281, "PhoenixMotorControlDevRef"=w43) -> ("error out"=w49:errorcluster, "PhoenixMotorControlDevRef"=w50:T12)  [unwired: 6 in]
  n74 = call <vilib>:"CTRE_Phoenix_MotorControl_SetStatusFramePeriod_Enhanced.vi"("error in (no error)"=w298, "periodMs"=w282, "Status Frame"=w281, "PhoenixMotorControlDevRef"=w297) -> ("error out"=w278:errorcluster, "PhoenixMotorControlDevRef"=w277:T12)  [unwired: 6 in]
  n75 = call <vilib>:"CTRE_Phoenix_MotorControl_SetStatusFramePeriod_Enhanced.vi"("error in (no error)"=w284, "periodMs"=w282, "Status Frame"=w281, "PhoenixMotorControlDevRef"=w283) -> ("error out"=w264:errorcluster, "PhoenixMotorControlDevRef"=w263:T12)  [unwired: 6 in]
  n76 = call <vilib>:"CTRE_Phoenix_MotorControl_SetStatusFramePeriod_Enhanced.vi"("error in (no error)"=w296, "periodMs"=w282, "Status Frame"=w281, "PhoenixMotorControlDevRef"=w295) -> ("error out"=w276:errorcluster, "PhoenixMotorControlDevRef"=w275:T12)  [unwired: 6 in]
  n77 = call <vilib>:"CTRE_Phoenix_MotorControl_SetStatusFramePeriod_Enhanced.vi"("error in (no error)"=w286, "periodMs"=w282, "Status Frame"=w281, "PhoenixMotorControlDevRef"=w285) -> ("error out"=w266:errorcluster, "PhoenixMotorControlDevRef"=w265:T12)  [unwired: 6 in]
  n78 = call <vilib>:"CTRE_Phoenix_MotorControl_SetStatusFramePeriod_Enhanced.vi"("error in (no error)"=w294, "periodMs"=150, "Status Frame"=w281, "PhoenixMotorControlDevRef"=w293) -> ("error out"=w274:errorcluster, "PhoenixMotorControlDevRef"=w273:T12)  [unwired: 6 in]
  n79 = call <vilib>:"CTRE_Phoenix_MotorControl_SetStatusFramePeriod_Enhanced.vi"("error in (no error)"=w288, "periodMs"=w282, "Status Frame"=w281, "PhoenixMotorControlDevRef"=w287) -> ("error out"=w268:errorcluster, "PhoenixMotorControlDevRef"=w267:T12)  [unwired: 6 in]
  n80 = call <vilib>:"CTRE_Phoenix_MotorControl_SetStatusFramePeriod_Enhanced.vi"("error in (no error)"=w300, "periodMs"=w282, "Status Frame"=w281, "PhoenixMotorControlDevRef"=w299) -> ("error out"=w280:errorcluster, "PhoenixMotorControlDevRef"=w279:T12)  [unwired: 6 in]
  n81 = call <vilib>:"CTRE_Phoenix_MotorControl_SetStatusFramePeriod_Enhanced.vi"("error in (no error)"=w292, "periodMs"=w282, "Status Frame"=w281, "PhoenixMotorControlDevRef"=w291) -> ("error out"=w272:errorcluster, "PhoenixMotorControlDevRef"=w271:T12)  [unwired: 6 in]
  n82 = call <vilib>:"CTRE_Phoenix_MotorControl_SetStatusFramePeriod_Enhanced.vi"("error in (no error)"=w290, "periodMs"=w282, "Status Frame"=w281, "PhoenixMotorControlDevRef"=w289) -> ("error out"=w270:errorcluster, "PhoenixMotorControlDevRef"=w269:T12)  [unwired: 6 in]
  n83 = call <vilib>:"CTRE_Phoenix_MotorControl_SetStatusFramePeriod_Enhanced.vi"("error in (no error)"=w51, "periodMs"=w262, "Status Frame"=w261, "PhoenixMotorControlDevRef"=w52) -> ("error out"=w58:errorcluster, "PhoenixMotorControlDevRef"=w59:T12)  [unwired: 6 in]
  n84 = call <vilib>:"CTRE_Phoenix_MotorControl_SetStatusFramePeriod_Enhanced.vi"("error in (no error)"=w53, "periodMs"=w262, "Status Frame"=w261, "PhoenixMotorControlDevRef"=w54) -> ("error out"=w60:errorcluster, "PhoenixMotorControlDevRef"=w61:T12)  [unwired: 6 in]
  n85 = call <vilib>:"CTRE_Phoenix_MotorControl_SetStatusFramePeriod_Enhanced.vi"("error in (no error)"=w48, "periodMs"=w262, "Status Frame"=w261, "PhoenixMotorControlDevRef"=w15) -> ("error out"=w55:errorcluster, "PhoenixMotorControlDevRef"=w14:T12)  [unwired: 6 in]
  n86 = call <vilib>:"CTRE_Phoenix_MotorControl_SetStatusFramePeriod_Enhanced.vi"("error in (no error)"=w49, "periodMs"=w262, "Status Frame"=w261, "PhoenixMotorControlDevRef"=w50) -> ("error out"=w56:errorcluster, "PhoenixMotorControlDevRef"=w57:T12)  [unwired: 6 in]
  n87 = call <vilib>:"CTRE_Phoenix_MotorControl_SetStatusFramePeriod_Enhanced.vi"("error in (no error)"=w278, "periodMs"=w262, "Status Frame"=w261, "PhoenixMotorControlDevRef"=w277) -> ("error out"=w258:errorcluster, "PhoenixMotorControlDevRef"=w257:T12)  [unwired: 6 in]
  n88 = call <vilib>:"CTRE_Phoenix_MotorControl_SetStatusFramePeriod_Enhanced.vi"("error in (no error)"=w268, "periodMs"=w262, "Status Frame"=w261, "PhoenixMotorControlDevRef"=w267) -> ("error out"=w248:errorcluster, "PhoenixMotorControlDevRef"=w247:T12)  [unwired: 6 in]
  n89 = call <vilib>:"CTRE_Phoenix_MotorControl_SetStatusFramePeriod_Enhanced.vi"("error in (no error)"=w276, "periodMs"=w262, "Status Frame"=w261, "PhoenixMotorControlDevRef"=w275) -> ("error out"=w254:errorcluster, "PhoenixMotorControlDevRef"=w253:T12)  [unwired: 6 in]
  n90 = call <vilib>:"CTRE_Phoenix_MotorControl_SetStatusFramePeriod_Enhanced.vi"("error in (no error)"=w264, "periodMs"=w262, "Status Frame"=w261, "PhoenixMotorControlDevRef"=w263) -> ("error out"=w244:errorcluster, "PhoenixMotorControlDevRef"=w243:T12)  [unwired: 6 in]
  n91 = call <vilib>:"CTRE_Phoenix_MotorControl_SetStatusFramePeriod_Enhanced.vi"("error in (no error)"=w280, "periodMs"=w262, "Status Frame"=w261, "PhoenixMotorControlDevRef"=w279) -> ("error out"=w260:errorcluster, "PhoenixMotorControlDevRef"=w259:T12)  [unwired: 6 in]
  n92 = call <vilib>:"CTRE_Phoenix_MotorControl_SetStatusFramePeriod_Enhanced.vi"("error in (no error)"=w266, "periodMs"=w262, "Status Frame"=w261, "PhoenixMotorControlDevRef"=w265) -> ("error out"=w246:errorcluster, "PhoenixMotorControlDevRef"=w245:T12)  [unwired: 6 in]
  n93 = call <vilib>:"CTRE_Phoenix_MotorControl_SetStatusFramePeriod_Enhanced.vi"("error in (no error)"=w274, "periodMs"=w262, "Status Frame"=w261, "PhoenixMotorControlDevRef"=w273) -> ("error out"=w256:errorcluster, "PhoenixMotorControlDevRef"=w255:T12)  [unwired: 6 in]
  n94 = call <vilib>:"CTRE_Phoenix_MotorControl_SetStatusFramePeriod_Enhanced.vi"("error in (no error)"=w272, "periodMs"=w262, "Status Frame"=w261, "PhoenixMotorControlDevRef"=w271) -> ("error out"=w252:errorcluster, "PhoenixMotorControlDevRef"=w251:T12)  [unwired: 6 in]
  n95 = call <vilib>:"CTRE_Phoenix_MotorControl_SetStatusFramePeriod_Enhanced.vi"("error in (no error)"=w270, "periodMs"=w262, "Status Frame"=w261, "PhoenixMotorControlDevRef"=w269) -> ("error out"=w250:errorcluster, "PhoenixMotorControlDevRef"=w249:T12)  [unwired: 6 in]
  n96 = call-poly <vilib>:"NT Write Value.vi"("String Array"=string[] ["Alternative 1", "Alternative 2"], "Name"="Auto List") -> ()  [unwired: 9 in, 1 out]
  n97 = call <vilib>:"CTRE_Phoenix_MotorControl_SetStatusFramePeriod_Enhanced.vi"("error in (no error)"=w60, "periodMs"=w242, "Status Frame"=w241, "PhoenixMotorControlDevRef"=w61) -> ("error out"=w94:errorcluster, "PhoenixMotorControlDevRef"=w93:T12)  [unwired: 6 in]
  n98 = call <vilib>:"CTRE_Phoenix_MotorControl_SetStatusFramePeriod_Enhanced.vi"("error in (no error)"=w55, "periodMs"=w242, "Status Frame"=w241, "PhoenixMotorControlDevRef"=w14) -> ("error out"=w62:errorcluster, "PhoenixMotorControlDevRef"=w13:T12)  [unwired: 6 in]
  n99 = call <vilib>:"CTRE_Phoenix_MotorControl_SetStatusFramePeriod_Enhanced.vi"("error in (no error)"=w58, "periodMs"=w242, "Status Frame"=w241, "PhoenixMotorControlDevRef"=w59) -> ("error out"=w95:errorcluster, "PhoenixMotorControlDevRef"=w96:T12)  [unwired: 6 in]
  n100 = call <vilib>:"CTRE_Phoenix_MotorControl_SetStatusFramePeriod_Enhanced.vi"("error in (no error)"=w56, "periodMs"=w242, "Status Frame"=w241, "PhoenixMotorControlDevRef"=w57) -> ("error out"=w63:errorcluster, "PhoenixMotorControlDevRef"=w64:T12)  [unwired: 6 in]
  n101 = call <vilib>:"CTRE_Phoenix_MotorControl_SetStatusFramePeriod_Enhanced.vi"("error in (no error)"=w258, "periodMs"=w242, "Status Frame"=w241, "PhoenixMotorControlDevRef"=w257) -> ("error out"=w236:errorcluster, "PhoenixMotorControlDevRef"=w235:T12)  [unwired: 6 in]
  n102 = call <vilib>:"CTRE_Phoenix_MotorControl_SetStatusFramePeriod_Enhanced.vi"("error in (no error)"=w254, "periodMs"=w242, "Status Frame"=w241, "PhoenixMotorControlDevRef"=w253) -> ("error out"=w234:errorcluster, "PhoenixMotorControlDevRef"=w233:T12)  [unwired: 6 in]
  n103 = call <vilib>:"CTRE_Phoenix_MotorControl_SetStatusFramePeriod_Enhanced.vi"("error in (no error)"=w248, "periodMs"=w242, "Status Frame"=w241, "PhoenixMotorControlDevRef"=w247) -> ("error out"=w198:errorcluster, "PhoenixMotorControlDevRef"=w197:T12)  [unwired: 6 in]
  n104 = call <vilib>:"CTRE_Phoenix_MotorControl_SetStatusFramePeriod_Enhanced.vi"("error in (no error)"=w244, "periodMs"=w242, "Status Frame"=w241, "PhoenixMotorControlDevRef"=w243) -> ("error out"=w154:errorcluster, "PhoenixMotorControlDevRef"=w153:T12)  [unwired: 6 in]
  n105 = call <vilib>:"CTRE_Phoenix_MotorControl_SetStatusFramePeriod_Enhanced.vi"("error in (no error)"=w260, "periodMs"=w242, "Status Frame"=w241, "PhoenixMotorControlDevRef"=w259) -> ("error out"=w238:errorcluster, "PhoenixMotorControlDevRef"=w237:T12)  [unwired: 6 in]
  n106 = call <vilib>:"CTRE_Phoenix_MotorControl_SetStatusFramePeriod_Enhanced.vi"("error in (no error)"=w252, "periodMs"=w242, "Status Frame"=w241, "PhoenixMotorControlDevRef"=w251) -> ("error out"=w196:errorcluster, "PhoenixMotorControlDevRef"=w195:T12)  [unwired: 6 in]
  n107 = call <vilib>:"CTRE_Phoenix_MotorControl_SetStatusFramePeriod_Enhanced.vi"("error in (no error)"=w246, "periodMs"=w242, "Status Frame"=w241, "PhoenixMotorControlDevRef"=w245) -> ("error out"=w156:errorcluster, "PhoenixMotorControlDevRef"=w155:T12)  [unwired: 6 in]
  n108 = call <vilib>:"CTRE_Phoenix_MotorControl_SetStatusFramePeriod_Enhanced.vi"("error in (no error)"=w256, "periodMs"=w242, "Status Frame"=w241, "PhoenixMotorControlDevRef"=w255) -> ("error out"=w202:errorcluster, "PhoenixMotorControlDevRef"=w201:T12)  [unwired: 6 in]
  n109 = call <vilib>:"CTRE_Phoenix_MotorControl_SetStatusFramePeriod_Enhanced.vi"("error in (no error)"=w250, "periodMs"=w242, "Status Frame"=w241, "PhoenixMotorControlDevRef"=w249) -> ("error out"=w200:errorcluster, "PhoenixMotorControlDevRef"=w199:T12)  [unwired: 6 in]
  n110 = call <vilib>:"CTRE_Phoenix_MotorControl_SetStatusFramePeriod_Enhanced.vi"("error in (no error)"=w94, "periodMs"=w132, "Status Frame"=w131, "PhoenixMotorControlDevRef"=w93) -> ("error out"=w85:errorcluster, "PhoenixMotorControlDevRef"=w86:T12)  [unwired: 6 in]
  n111 = call <vilib>:"CTRE_Phoenix_MotorControl_SetStatusFramePeriod_Enhanced.vi"("error in (no error)"=w62, "periodMs"=w132, "Status Frame"=w131, "PhoenixMotorControlDevRef"=w13) -> ("error out"=w65:errorcluster, "PhoenixMotorControlDevRef"=w12:T12)  [unwired: 6 in]
  n112 = call <vilib>:"CTRE_Phoenix_MotorControl_SetStatusFramePeriod_Enhanced.vi"("error in (no error)"=w63, "periodMs"=w132, "Status Frame"=w131, "PhoenixMotorControlDevRef"=w64) -> ("error out"=w66:errorcluster, "PhoenixMotorControlDevRef"=w67:T12)  [unwired: 6 in]
  n113 = call <vilib>:"CTRE_Phoenix_MotorControl_SetStatusFramePeriod_Enhanced.vi"("error in (no error)"=w95, "periodMs"=w132, "Status Frame"=w131, "PhoenixMotorControlDevRef"=w96) -> ("error out"=w77:errorcluster, "PhoenixMotorControlDevRef"=w78:T12)  [unwired: 6 in]
  n114 = call <vilib>:"CTRE_Phoenix_MotorControl_SetStatusFramePeriod_Enhanced.vi"("error in (no error)"=w236, "periodMs"=w132, "Status Frame"=w131, "PhoenixMotorControlDevRef"=w235) -> ("error out"=w230:errorcluster, "PhoenixMotorControlDevRef"=w229:T12)  [unwired: 6 in]
  n115 = call <vilib>:"CTRE_Phoenix_MotorControl_SetStatusFramePeriod_Enhanced.vi"("error in (no error)"=w238, "periodMs"=w132, "Status Frame"=w131, "PhoenixMotorControlDevRef"=w237) -> ("error out"=w232:errorcluster, "PhoenixMotorControlDevRef"=w231:T12)  [unwired: 6 in]
  n116 = call <vilib>:"CTRE_Phoenix_MotorControl_SetStatusFramePeriod_Enhanced.vi"("error in (no error)"=w196, "periodMs"=w132, "Status Frame"=w131, "PhoenixMotorControlDevRef"=w195) -> ("error out"=w192:errorcluster, "PhoenixMotorControlDevRef"=w191:T12)  [unwired: 6 in]
  n117 = call <vilib>:"CTRE_Phoenix_MotorControl_SetStatusFramePeriod_Enhanced.vi"("error in (no error)"=w198, "periodMs"=w132, "Status Frame"=w131, "PhoenixMotorControlDevRef"=w197) -> ("error out"=w130:errorcluster, "PhoenixMotorControlDevRef"=w129:T12)  [unwired: 6 in]
  n118 = call <vilib>:"CTRE_Phoenix_MotorControl_SetStatusFramePeriod_Enhanced.vi"("error in (no error)"=w200, "periodMs"=w132, "Status Frame"=w131, "PhoenixMotorControlDevRef"=w199) -> ("error out"=w190:errorcluster, "PhoenixMotorControlDevRef"=w189:T12)  [unwired: 6 in]
  n119 = call <vilib>:"CTRE_Phoenix_MotorControl_SetStatusFramePeriod_Enhanced.vi"("error in (no error)"=w202, "periodMs"=w132, "Status Frame"=w131, "PhoenixMotorControlDevRef"=w201) -> ("error out"=w194:errorcluster, "PhoenixMotorControlDevRef"=w193:T12)  [unwired: 6 in]
  n120 = call <vilib>:"CTRE_Phoenix_MotorControl_SetStatusFramePeriod_Enhanced.vi"("error in (no error)"=w234, "periodMs"=w132, "Status Frame"=w131, "PhoenixMotorControlDevRef"=w233) -> ("error out"=w228:errorcluster, "PhoenixMotorControlDevRef"=w227:T12)  [unwired: 6 in]
  n121 = call <vilib>:"CTRE_Phoenix_MotorControl_SetStatusFramePeriod_Enhanced.vi"("error in (no error)"=w154, "periodMs"=w132, "Status Frame"=w131, "PhoenixMotorControlDevRef"=w153) -> ("error out"=w150:errorcluster, "PhoenixMotorControlDevRef"=w149:T12)  [unwired: 6 in]
  n122 = call <vilib>:"CTRE_Phoenix_MotorControl_SetStatusFramePeriod_Enhanced.vi"("error in (no error)"=w156, "periodMs"=w132, "Status Frame"=w131, "PhoenixMotorControlDevRef"=w155) -> ("error out"=w152:errorcluster, "PhoenixMotorControlDevRef"=w151:T12)  [unwired: 6 in]
  n123 = call <vilib>:"Color Sensor V3 Open.vi"("I2C Bus"=i2c_bus."I2C On-Board") -> ("error out"=w412:errorcluster, "ColorSensorDevRef"=w411:T16)  [unwired: 9 in]
  n124 = call <vilib>:"CTRE_Phoenix_MotorControl_SetStatusFramePeriod_Enhanced.vi"("error in (no error)"=w85, "periodMs"=w128, "Status Frame"=w127, "PhoenixMotorControlDevRef"=w86) -> ("error out"=w87:errorcluster, "PhoenixMotorControlDevRef"=w88:T12)  [unwired: 6 in]
  n125 = call <vilib>:"CTRE_Phoenix_MotorControl_SetStatusFramePeriod_Enhanced.vi"("error in (no error)"=w65, "periodMs"=w128, "Status Frame"=w127, "PhoenixMotorControlDevRef"=w12) -> ("error out"=w68:errorcluster, "PhoenixMotorControlDevRef"=w11:T12)  [unwired: 6 in]
  n126 = call <vilib>:"CTRE_Phoenix_MotorControl_SetStatusFramePeriod_Enhanced.vi"("error in (no error)"=w66, "periodMs"=w128, "Status Frame"=w127, "PhoenixMotorControlDevRef"=w67) -> ("error out"=w69:errorcluster, "PhoenixMotorControlDevRef"=w70:T12)  [unwired: 6 in]
  n127 = call <vilib>:"CTRE_Phoenix_MotorControl_SetStatusFramePeriod_Enhanced.vi"("error in (no error)"=w77, "periodMs"=w128, "Status Frame"=w127, "PhoenixMotorControlDevRef"=w78) -> ("error out"=w79:errorcluster, "PhoenixMotorControlDevRef"=w80:T12)  [unwired: 6 in]
  n128 = call <vilib>:"CTRE_Phoenix_MotorControl_SetStatusFramePeriod_Enhanced.vi"("error in (no error)"=w232, "periodMs"=w128, "Status Frame"=w127, "PhoenixMotorControlDevRef"=w231) -> ("error out"=w226:errorcluster, "PhoenixMotorControlDevRef"=w225:T12)  [unwired: 6 in]
  n129 = call <vilib>:"CTRE_Phoenix_MotorControl_SetStatusFramePeriod_Enhanced.vi"("error in (no error)"=w230, "periodMs"=w128, "Status Frame"=w127, "PhoenixMotorControlDevRef"=w229) -> ("error out"=w224:errorcluster, "PhoenixMotorControlDevRef"=w223:T12)  [unwired: 6 in]
  n130 = call <vilib>:"CTRE_Phoenix_MotorControl_SetStatusFramePeriod_Enhanced.vi"("error in (no error)"=w192, "periodMs"=w128, "Status Frame"=w127, "PhoenixMotorControlDevRef"=w191) -> ("error out"=w186:errorcluster, "PhoenixMotorControlDevRef"=w185:T12)  [unwired: 6 in]
  n131 = call <vilib>:"CTRE_Phoenix_MotorControl_SetStatusFramePeriod_Enhanced.vi"("error in (no error)"=w194, "periodMs"=w128, "Status Frame"=w127, "PhoenixMotorControlDevRef"=w193) -> ("error out"=w188:errorcluster, "PhoenixMotorControlDevRef"=w187:T12)  [unwired: 6 in]
  n132 = call <vilib>:"CTRE_Phoenix_MotorControl_SetStatusFramePeriod_Enhanced.vi"("error in (no error)"=w228, "periodMs"=w128, "Status Frame"=w127, "PhoenixMotorControlDevRef"=w227) -> ("error out"=w222:errorcluster, "PhoenixMotorControlDevRef"=w221:T12)  [unwired: 6 in]
  n133 = call <vilib>:"CTRE_Phoenix_MotorControl_SetStatusFramePeriod_Enhanced.vi"("error in (no error)"=w130, "periodMs"=w128, "Status Frame"=w127, "PhoenixMotorControlDevRef"=w129) -> ("error out"=w182:errorcluster, "PhoenixMotorControlDevRef"=w181:T12)  [unwired: 6 in]
  n134 = call <vilib>:"CTRE_Phoenix_MotorControl_SetStatusFramePeriod_Enhanced.vi"("error in (no error)"=w152, "periodMs"=w128, "Status Frame"=w127, "PhoenixMotorControlDevRef"=w151) -> ("error out"=w148:errorcluster, "PhoenixMotorControlDevRef"=w147:T12)  [unwired: 6 in]
  n135 = call <vilib>:"CTRE_Phoenix_MotorControl_SetStatusFramePeriod_Enhanced.vi"("error in (no error)"=w190, "periodMs"=w128, "Status Frame"=w127, "PhoenixMotorControlDevRef"=w189) -> ("error out"=w184:errorcluster, "PhoenixMotorControlDevRef"=w183:T12)  [unwired: 6 in]
  n136 = call <vilib>:"CTRE_Phoenix_MotorControl_SetStatusFramePeriod_Enhanced.vi"("error in (no error)"=w150, "periodMs"=w128, "Status Frame"=w127, "PhoenixMotorControlDevRef"=w149) -> ("error out"=w146:errorcluster, "PhoenixMotorControlDevRef"=w145:T12)  [unwired: 6 in]
  n137 = call <vilib>:"Color Sensor V3 RefNum Registry Set.vi"("error in (no error)"=w412, "refnum name"="ColorSensor", "ColorSensorDevRef"=w411) -> ()  [unwired: 7 in, 2 out]
  n138 = call <vilib>:"CTRE_Phoenix_MotorControl_SetStatusFramePeriod_Enhanced.vi"("error in (no error)"=w87, "periodMs"=w126, "Status Frame"=w125, "PhoenixMotorControlDevRef"=w88) -> ("error out"=w89:errorcluster, "PhoenixMotorControlDevRef"=w90:T12)  [unwired: 6 in]
  n139 = call <vilib>:"CTRE_Phoenix_MotorControl_SetStatusFramePeriod_Enhanced.vi"("error in (no error)"=w68, "periodMs"=w126, "Status Frame"=w125, "PhoenixMotorControlDevRef"=w11) -> ("error out"=w71:errorcluster, "PhoenixMotorControlDevRef"=w10:T12)  [unwired: 6 in]
  n140 = call <vilib>:"CTRE_Phoenix_MotorControl_SetStatusFramePeriod_Enhanced.vi"("error in (no error)"=w69, "periodMs"=w126, "Status Frame"=w125, "PhoenixMotorControlDevRef"=w70) -> ("error out"=w72:errorcluster, "PhoenixMotorControlDevRef"=w73:T12)  [unwired: 6 in]
  n141 = call <vilib>:"CTRE_Phoenix_MotorControl_SetStatusFramePeriod_Enhanced.vi"("error in (no error)"=w79, "periodMs"=w126, "Status Frame"=w125, "PhoenixMotorControlDevRef"=w80) -> ("error out"=w81:errorcluster, "PhoenixMotorControlDevRef"=w82:T12)  [unwired: 6 in]
  n142 = call <vilib>:"CTRE_Phoenix_MotorControl_SetStatusFramePeriod_Enhanced.vi"("error in (no error)"=w226, "periodMs"=w126, "Status Frame"=w125, "PhoenixMotorControlDevRef"=w225) -> ("error out"=w220:errorcluster, "PhoenixMotorControlDevRef"=w219:T12)  [unwired: 6 in]
  n143 = call <vilib>:"CTRE_Phoenix_MotorControl_SetStatusFramePeriod_Enhanced.vi"("error in (no error)"=w186, "periodMs"=w126, "Status Frame"=w125, "PhoenixMotorControlDevRef"=w185) -> ("error out"=w178:errorcluster, "PhoenixMotorControlDevRef"=w177:T12)  [unwired: 6 in]
  n144 = call <vilib>:"CTRE_Phoenix_MotorControl_SetStatusFramePeriod_Enhanced.vi"("error in (no error)"=w146, "periodMs"=w126, "Status Frame"=w125, "PhoenixMotorControlDevRef"=w145) -> ("error out"=w142:errorcluster, "PhoenixMotorControlDevRef"=w141:T12)  [unwired: 6 in]
  n145 = call <vilib>:"CTRE_Phoenix_MotorControl_SetStatusFramePeriod_Enhanced.vi"("error in (no error)"=w224, "periodMs"=w126, "Status Frame"=w125, "PhoenixMotorControlDevRef"=w223) -> ("error out"=w218:errorcluster, "PhoenixMotorControlDevRef"=w217:T12)  [unwired: 6 in]
  n146 = call <vilib>:"CTRE_Phoenix_MotorControl_SetStatusFramePeriod_Enhanced.vi"("error in (no error)"=w148, "periodMs"=w126, "Status Frame"=w125, "PhoenixMotorControlDevRef"=w147) -> ("error out"=w144:errorcluster, "PhoenixMotorControlDevRef"=w143:T12)  [unwired: 6 in]
  n147 = call <vilib>:"CTRE_Phoenix_MotorControl_SetStatusFramePeriod_Enhanced.vi"("error in (no error)"=w184, "periodMs"=w126, "Status Frame"=w125, "PhoenixMotorControlDevRef"=w183) -> ("error out"=w176:errorcluster, "PhoenixMotorControlDevRef"=w175:T12)  [unwired: 6 in]
  n148 = call <vilib>:"CTRE_Phoenix_MotorControl_SetStatusFramePeriod_Enhanced.vi"("error in (no error)"=w222, "periodMs"=w126, "Status Frame"=w125, "PhoenixMotorControlDevRef"=w221) -> ("error out"=w216:errorcluster, "PhoenixMotorControlDevRef"=w215:T12)  [unwired: 6 in]
  n149 = call <vilib>:"CTRE_Phoenix_MotorControl_SetStatusFramePeriod_Enhanced.vi"("error in (no error)"=w188, "periodMs"=w126, "Status Frame"=w125, "PhoenixMotorControlDevRef"=w187) -> ("error out"=w180:errorcluster, "PhoenixMotorControlDevRef"=w179:T12)  [unwired: 6 in]
  n150 = call <vilib>:"CTRE_Phoenix_MotorControl_SetStatusFramePeriod_Enhanced.vi"("error in (no error)"=w182, "periodMs"=w126, "Status Frame"=w125, "PhoenixMotorControlDevRef"=w181) -> ("error out"=w174:errorcluster, "PhoenixMotorControlDevRef"=w173:T12)  [unwired: 6 in]
  n151 = call <vilib>:"CTRE_Phoenix_MotorControl_SetStatusFramePeriod_Enhanced.vi"("error in (no error)"=w71, "periodMs"=w124, "Status Frame"=w123, "PhoenixMotorControlDevRef"=w10) -> ("error out"=w74:errorcluster, "PhoenixMotorControlDevRef"=w9:T12)  [unwired: 6 in]
  n152 = call <vilib>:"CTRE_Phoenix_MotorControl_SetStatusFramePeriod_Enhanced.vi"("error in (no error)"=w89, "periodMs"=w124, "Status Frame"=w123, "PhoenixMotorControlDevRef"=w90) -> ("error out"=w91:errorcluster, "PhoenixMotorControlDevRef"=w92:T12)  [unwired: 6 in]
  n153 = call <vilib>:"CTRE_Phoenix_MotorControl_SetStatusFramePeriod_Enhanced.vi"("error in (no error)"=w220, "periodMs"=w124, "Status Frame"=w123, "PhoenixMotorControlDevRef"=w219) -> ("error out"=w214:errorcluster, "PhoenixMotorControlDevRef"=w213:T12)  [unwired: 6 in]
  n154 = call <vilib>:"CTRE_Phoenix_MotorControl_SetStatusFramePeriod_Enhanced.vi"("error in (no error)"=w72, "periodMs"=w124, "Status Frame"=w123, "PhoenixMotorControlDevRef"=w73) -> ("error out"=w75:errorcluster, "PhoenixMotorControlDevRef"=w76:T12)  [unwired: 6 in]
  n155 = call <vilib>:"CTRE_Phoenix_MotorControl_SetStatusFramePeriod_Enhanced.vi"("error in (no error)"=w81, "periodMs"=w124, "Status Frame"=w123, "PhoenixMotorControlDevRef"=w82) -> ("error out"=w83:errorcluster, "PhoenixMotorControlDevRef"=w84:T12)  [unwired: 6 in]
  n156 = call <vilib>:"CTRE_Phoenix_MotorControl_SetStatusFramePeriod_Enhanced.vi"("error in (no error)"=w176, "periodMs"=w124, "Status Frame"=w123, "PhoenixMotorControlDevRef"=w175) -> ("error out"=w168:errorcluster, "PhoenixMotorControlDevRef"=w167:T12)  [unwired: 6 in]
  n157 = call <vilib>:"CTRE_Phoenix_MotorControl_SetStatusFramePeriod_Enhanced.vi"("error in (no error)"=w218, "periodMs"=w124, "Status Frame"=w123, "PhoenixMotorControlDevRef"=w217) -> ("error out"=w212:errorcluster, "PhoenixMotorControlDevRef"=w211:T12)  [unwired: 6 in]
  n158 = call <vilib>:"CTRE_Phoenix_MotorControl_SetStatusFramePeriod_Enhanced.vi"("error in (no error)"=w144, "periodMs"=w124, "Status Frame"=w123, "PhoenixMotorControlDevRef"=w143) -> ("error out"=w140:errorcluster, "PhoenixMotorControlDevRef"=w139:T12)  [unwired: 6 in]
  n159 = call <vilib>:"CTRE_Phoenix_MotorControl_SetStatusFramePeriod_Enhanced.vi"("error in (no error)"=w178, "periodMs"=w124, "Status Frame"=w123, "PhoenixMotorControlDevRef"=w177) -> ("error out"=w170:errorcluster, "PhoenixMotorControlDevRef"=w169:T12)  [unwired: 6 in]
  n160 = call <vilib>:"CTRE_Phoenix_MotorControl_SetStatusFramePeriod_Enhanced.vi"("error in (no error)"=w142, "periodMs"=w124, "Status Frame"=w123, "PhoenixMotorControlDevRef"=w141) -> ("error out"=w138:errorcluster, "PhoenixMotorControlDevRef"=w137:T12)  [unwired: 6 in]
  n161 = call <vilib>:"CTRE_Phoenix_MotorControl_SetStatusFramePeriod_Enhanced.vi"("error in (no error)"=w180, "periodMs"=w124, "Status Frame"=w123, "PhoenixMotorControlDevRef"=w179) -> ("error out"=w172:errorcluster, "PhoenixMotorControlDevRef"=w171:T12)  [unwired: 6 in]
  n162 = call <vilib>:"CTRE_Phoenix_MotorControl_SetStatusFramePeriod_Enhanced.vi"("error in (no error)"=w216, "periodMs"=w124, "Status Frame"=w123, "PhoenixMotorControlDevRef"=w215) -> ("error out"=w210:errorcluster, "PhoenixMotorControlDevRef"=w209:T12)  [unwired: 6 in]
  n163 = call <vilib>:"CTRE_Phoenix_MotorControl_SetStatusFramePeriod_Enhanced.vi"("error in (no error)"=w174, "periodMs"=w124, "Status Frame"=w123, "PhoenixMotorControlDevRef"=w173) -> ("error out"=w166:errorcluster, "PhoenixMotorControlDevRef"=w165:T12)  [unwired: 6 in]
  n164 = call <vilib>:"CTRE_Phoenix_Pigeon2_Open.vi"("Device Number"=u8 20) -> ("error out"=w107:errorcluster, "PigeonIMUDevRef"=w108:T18)  [unwired: 9 in]
  n165 = call <vilib>:"CTRE_Phoenix_MotorControl_SetStatusFramePeriod_Enhanced.vi"("error in (no error)"=w74, "periodMs"=w122, "Status Frame"=w121, "PhoenixMotorControlDevRef"=w9) -> ("error out"=w19:errorcluster, "PhoenixMotorControlDevRef"=w18:T12)  [unwired: 6 in]
  n166 = call <vilib>:"CTRE_Phoenix_MotorControl_SetStatusFramePeriod_Enhanced.vi"("error in (no error)"=w91, "periodMs"=w122, "Status Frame"=w121, "PhoenixMotorControlDevRef"=w92) -> ("error out"=w25:errorcluster, "PhoenixMotorControlDevRef"=w24:T12)  [unwired: 6 in]
  n167 = call <vilib>:"CTRE_Phoenix_MotorControl_SetStatusFramePeriod_Enhanced.vi"("error in (no error)"=w75, "periodMs"=w122, "Status Frame"=w121, "PhoenixMotorControlDevRef"=w76) -> ("error out"=w21:errorcluster, "PhoenixMotorControlDevRef"=w20:T12)  [unwired: 6 in]
  n168 = call <vilib>:"CTRE_Phoenix_MotorControl_SetStatusFramePeriod_Enhanced.vi"("error in (no error)"=w214, "periodMs"=w122, "Status Frame"=w121, "PhoenixMotorControlDevRef"=w213) -> ("error out"=w207:errorcluster, "PhoenixMotorControlDevRef"=w208:T12)  [unwired: 6 in]
  n169 = call <vilib>:"CTRE_Phoenix_MotorControl_SetStatusFramePeriod_Enhanced.vi"("error in (no error)"=w83, "periodMs"=w122, "Status Frame"=w121, "PhoenixMotorControlDevRef"=w84) -> ("error out"=w23:errorcluster, "PhoenixMotorControlDevRef"=w22:T12)  [unwired: 6 in]
  n170 = call <vilib>:"CTRE_Phoenix_MotorControl_SetStatusFramePeriod_Enhanced.vi"("error in (no error)"=w168, "periodMs"=w122, "Status Frame"=w121, "PhoenixMotorControlDevRef"=w167) -> ("error out"=w159:errorcluster, "PhoenixMotorControlDevRef"=w160:T12)  [unwired: 6 in]
  n171 = call <vilib>:"CTRE_Phoenix_MotorControl_SetStatusFramePeriod_Enhanced.vi"("error in (no error)"=w172, "periodMs"=w122, "Status Frame"=w121, "PhoenixMotorControlDevRef"=w171) -> ("error out"=w163:errorcluster, "PhoenixMotorControlDevRef"=w164:T12)  [unwired: 6 in]
  n172 = call <vilib>:"CTRE_Phoenix_MotorControl_SetStatusFramePeriod_Enhanced.vi"("error in (no error)"=w212, "periodMs"=w122, "Status Frame"=w121, "PhoenixMotorControlDevRef"=w211) -> ("error out"=w205:errorcluster, "PhoenixMotorControlDevRef"=w206:T12)  [unwired: 6 in]
  n173 = call <vilib>:"CTRE_Phoenix_MotorControl_SetStatusFramePeriod_Enhanced.vi"("error in (no error)"=w138, "periodMs"=w122, "Status Frame"=w121, "PhoenixMotorControlDevRef"=w137) -> ("error out"=w133:errorcluster, "PhoenixMotorControlDevRef"=w134:T12)  [unwired: 6 in]
  n174 = call <vilib>:"CTRE_Phoenix_MotorControl_SetStatusFramePeriod_Enhanced.vi"("error in (no error)"=w140, "periodMs"=w122, "Status Frame"=w121, "PhoenixMotorControlDevRef"=w139) -> ("error out"=w135:errorcluster, "PhoenixMotorControlDevRef"=w136:T12)  [unwired: 6 in]
  n175 = call <vilib>:"CTRE_Phoenix_MotorControl_SetStatusFramePeriod_Enhanced.vi"("error in (no error)"=w170, "periodMs"=w122, "Status Frame"=w121, "PhoenixMotorControlDevRef"=w169) -> ("error out"=w161:errorcluster, "PhoenixMotorControlDevRef"=w162:T12)  [unwired: 6 in]
  n176 = call <vilib>:"CTRE_Phoenix_MotorControl_SetStatusFramePeriod_Enhanced.vi"("error in (no error)"=w210, "periodMs"=w122, "Status Frame"=w121, "PhoenixMotorControlDevRef"=w209) -> ("error out"=w203:errorcluster, "PhoenixMotorControlDevRef"=w204:T12)  [unwired: 6 in]
  n177 = call <vilib>:"CTRE_Phoenix_MotorControl_SetStatusFramePeriod_Enhanced.vi"("error in (no error)"=w166, "periodMs"=w122, "Status Frame"=w121, "PhoenixMotorControlDevRef"=w165) -> ("error out"=w157:errorcluster, "PhoenixMotorControlDevRef"=w158:T12)  [unwired: 6 in]
  n178 = call <vilib>:"CTRE_Phoenix_Pigeon2_ConfigMountPoseYaw.vi"("error in"=w107, "Yaw"=90.0, "PigeonIMUDevRef"=w108) -> ("error out"=w105:errorcluster, "PigeonIMUDevRef 2"=w106:T18)  [unwired: 7 in]
  n179 = call <vilib>:"CTRE_PigeonIMU_RefNumRegistrySet.vi"("error in (no error)"=w105, "refnum name"="Pigeon", "PigeonIMUDevRef"=w106) -> ()  [unwired: 7 in, 2 out]
  n180 = call-poly <vilib>:"CTRE_Phoenix_MotorController_Get_TalonFX.vi"("PhoenixMotorControlDevRef"=w160, "error in"=w159) -> ("PhoenixMotorControlDevRef"=w305:T12, "error out"=w449:errorcluster)  [unwired: 10 in, 2 out]
  n181 = call-poly <vilib>:"CTRE_Phoenix_MotorController_Get_TalonFX.vi"("PhoenixMotorControlDevRef"=w20, "error in"=w21) -> ("PhoenixMotorControlDevRef"=w346:T12, "error out"=w358:errorcluster)  [unwired: 10 in, 2 out]
  n182 = call-poly <vilib>:"CTRE_Phoenix_MotorController_Get_TalonFX.vi"("PhoenixMotorControlDevRef"=w22, "error in"=w23) -> ("PhoenixMotorControlDevRef"=w354:T12, "error out"=w355:errorcluster)  [unwired: 10 in, 2 out]
  n183 = call-poly <vilib>:"CTRE_Phoenix_MotorController_Get_TalonFX.vi"("PhoenixMotorControlDevRef"=w24, "error in"=w25) -> ("PhoenixMotorControlDevRef"=w350:T12, "error out"=w351:errorcluster)  [unwired: 10 in, 2 out]
  n184 = call-poly <vilib>:"CTRE_Phoenix_MotorController_Get_TalonFX.vi"("PhoenixMotorControlDevRef"=w158, "error in"=w157) -> ("PhoenixMotorControlDevRef"=w441:T12, "error out"=w442:errorcluster)  [unwired: 10 in, 2 out]
  n185 = call-poly <vilib>:"CTRE_Phoenix_MotorController_Get_TalonFX.vi"("PhoenixMotorControlDevRef"=w136, "error in"=w135) -> ("PhoenixMotorControlDevRef"=w347:T12, "error out"=w306:errorcluster)  [unwired: 10 in, 2 out]
  n186 = call-poly <vilib>:"CTRE_Phoenix_MotorController_Get_TalonFX.vi"("PhoenixMotorControlDevRef"=w134, "error in"=w133) -> ("PhoenixMotorControlDevRef"=w307:T12, "error out"=w428:errorcluster)  [unwired: 10 in, 2 out]
  n187 = call-poly <vilib>:"CTRE_Phoenix_MotorController_Get_TalonFX.vi"("PhoenixMotorControlDevRef"=w18, "error in"=w19) -> ("PhoenixMotorControlDevRef"=w308:T12, "error out"=w361:errorcluster)  [unwired: 10 in, 2 out]
  n188 = call <vilib>:"CTRE_Phoenix_MotorControl_RefNumRegistrySet.vi"("error in (no error)"=w116, "refnum name"="Orange Front Drive", "PhoenixMotorControlDevRef"=w115) -> ()  [unwired: 7 in, 2 out]
  n189 = call <vilib>:"CTRE_Phoenix_MotorControl_RefNumRegistrySet.vi"("error in (no error)"=w111, "refnum name"="Blue Front Drive", "PhoenixMotorControlDevRef"=w112) -> ()  [unwired: 7 in, 2 out]
  n190 = call <vilib>:"CTRE_Phoenix_MotorControl_RefNumRegistrySet.vi"("error in (no error)"=w109, "refnum name"="Blue Back Drive", "PhoenixMotorControlDevRef"=w110) -> ()  [unwired: 7 in, 2 out]
  n191 = call <vilib>:"CTRE_Phoenix_MotorControl_RefNumRegistrySet.vi"("error in (no error)"=w207, "refnum name"="Elevate", "PhoenixMotorControlDevRef"=w208) -> ()  [unwired: 7 in, 2 out]
  n192 = call <vilib>:"CTRE_Phoenix_MotorControl_RefNumRegistrySet.vi"("error in (no error)"=w114, "refnum name"="Orange Back Drive", "PhoenixMotorControlDevRef"=w113) -> ()  [unwired: 7 in, 2 out]
  n193 = call <vilib>:"CTRE_Phoenix_MotorControl_RefNumRegistrySet.vi"("error in (no error)"=w205, "refnum name"="Reject", "PhoenixMotorControlDevRef"=w206) -> ()  [unwired: 7 in, 2 out]
  n194 = call <vilib>:"CTRE_Phoenix_MotorControl_RefNumRegistrySet.vi"("error in (no error)"=w203, "refnum name"="Intake", "PhoenixMotorControlDevRef"=w204) -> ()  [unwired: 7 in, 2 out]
  n195 = call <vilib>:"CTRE_Phoenix_MotorControl_RefNumRegistrySet.vi"("error in (no error)"=w163, "refnum name"="Shoot", "PhoenixMotorControlDevRef"=w164) -> ()  [unwired: 7 in, 2 out]
  n196 = call <vilib>:"CTRE_Phoenix_MotorControl_RefNumRegistrySet.vi"("error in (no error)"=w161, "refnum name"="Turret", "PhoenixMotorControlDevRef"=w162) -> ()  [unwired: 7 in, 2 out]
  n197 = call <vilib>:"CTRE_Phoenix_MotorControl_RefNumRegistrySet.vi"("error in (no error)"=w449, "refnum name"="Orange Back Turn", "PhoenixMotorControlDevRef"=w305) -> ()  [unwired: 7 in, 2 out]
  n198 = call <vilib>:"CTRE_Phoenix_MotorControl_RefNumRegistrySet.vi"("error in (no error)"=w358, "refnum name"="Orange Inside Climb", "PhoenixMotorControlDevRef"=w346) -> ()  [unwired: 7 in, 2 out]
  n199 = call <vilib>:"CTRE_Phoenix_MotorControl_RefNumRegistrySet.vi"("error in (no error)"=w355, "refnum name"="Blue Outside Climb", "PhoenixMotorControlDevRef"=w354) -> ()  [unwired: 7 in, 2 out]
  n200 = call <vilib>:"CTRE_Phoenix_MotorControl_RefNumRegistrySet.vi"("error in (no error)"=w351, "refnum name"="Blue Inside Climb", "PhoenixMotorControlDevRef"=w350) -> ()  [unwired: 7 in, 2 out]
  n201 = call <vilib>:"CTRE_Phoenix_MotorControl_RefNumRegistrySet.vi"("error in (no error)"=w442, "refnum name"="Orange Front Turn", "PhoenixMotorControlDevRef"=w441) -> ()  [unwired: 7 in, 2 out]
  n202 = call <vilib>:"CTRE_Phoenix_MotorControl_RefNumRegistrySet.vi"("error in (no error)"=w306, "refnum name"="Blue Front Turn", "PhoenixMotorControlDevRef"=w347) -> ()  [unwired: 7 in, 2 out]
  n203 = call <vilib>:"CTRE_Phoenix_MotorControl_RefNumRegistrySet.vi"("error in (no error)"=w428, "refnum name"="Blue Back Turn", "PhoenixMotorControlDevRef"=w307) -> ()  [unwired: 7 in, 2 out]
  n204 = call <vilib>:"CTRE_Phoenix_MotorControl_RefNumRegistrySet.vi"("error in (no error)"=w361, "refnum name"="Orange Outside Climb", "PhoenixMotorControlDevRef"=w308) -> ()  [unwired: 7 in, 2 out]
  n205 = call <vilib>:"CTRE_Phoenix_CANcoder_Open.vi"("Device Number"=u8 24) -> ("error out"=w117:errorcluster, "CTRE_CANcoder_DeviceRef"=w118:T20)  [unwired: 9 in]
  n206 = call <vilib>:"CTRE_Phoenix_CANcoder_Open.vi"("Device Number"=u8 21) -> ("error out"=w100:errorcluster, "CTRE_CANcoder_DeviceRef"=w101:T20)  [unwired: 9 in]
  n207 = call <vilib>:"CTRE_Phoenix_CANcoder_Open.vi"("Device Number"=u8 22) -> ("error out"=w103:errorcluster, "CTRE_CANcoder_DeviceRef"=w102:T20)  [unwired: 9 in]
  n208 = call <vilib>:"CTRE_Phoenix_CANcoder_Open.vi"("Device Number"=u8 23) -> ("error out"=w119:errorcluster, "CTRE_CANcoder_DeviceRef"=w120:T20)  [unwired: 9 in]
  n209 = call <vilib>:"CTRE_Phoenix_CANcoder_ConfigMagnetOffset.vi"("error in"=w100, "Magnet Offset (Degrees)"=0.0, "CTRE_CANcoder_DeviceRef"=w101) -> ("error out"=w99:errorcluster, "CTRE_CANcoder_DeviceRef"=w98:T20)  [unwired: 7 in]
  n210 = call <vilib>:"CTRE_Phoenix_CANcoder_RefNumRegistrySet.vi"("error in (no error)"=w117, "refnum name"="Blue Back Cancoder", "CTRE_CANcoder_DeviceRef"=w118) -> ()  [unwired: 7 in, 2 out]
  n211 = call <vilib>:"CTRE_Phoenix_CANcoder_RefNumRegistrySet.vi"("error in (no error)"=w99, "refnum name"="Orange Back Cancoder", "CTRE_CANcoder_DeviceRef"=w98) -> ()  [unwired: 7 in, 2 out]
  n212 = call <vilib>:"CTRE_Phoenix_CANcoder_RefNumRegistrySet.vi"("error in (no error)"=w103, "refnum name"="Orange Front Cancoder", "CTRE_CANcoder_DeviceRef"=w102) -> ()  [unwired: 7 in, 2 out]
  n213 = call <vilib>:"CTRE_Phoenix_CANcoder_RefNumRegistrySet.vi"("error in (no error)"=w119, "refnum name"="Blue Front Cancoder", "CTRE_CANcoder_DeviceRef"=w120) -> ()  [unwired: 7 in, 2 out]
  "error out" <- "error in"
